vi "tabs_test.vi"() -> ()   [LabVIEW 2015]
panel:
  in  "stop":bool
  in  "Tab Control 2":enum32{"DLTS", "CV", "IV"}(tab)
  in  "Numeric Control":dbl
  in  "Vertical Fill Slide":dbl(slide) scale=0.0..10.0
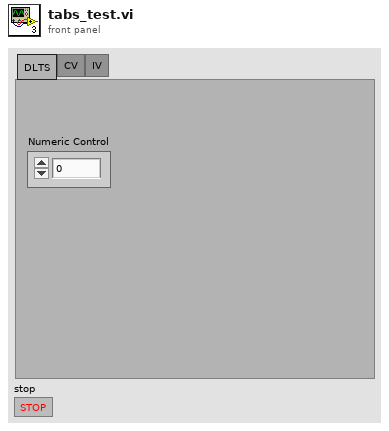
[diagram p1: front panel]
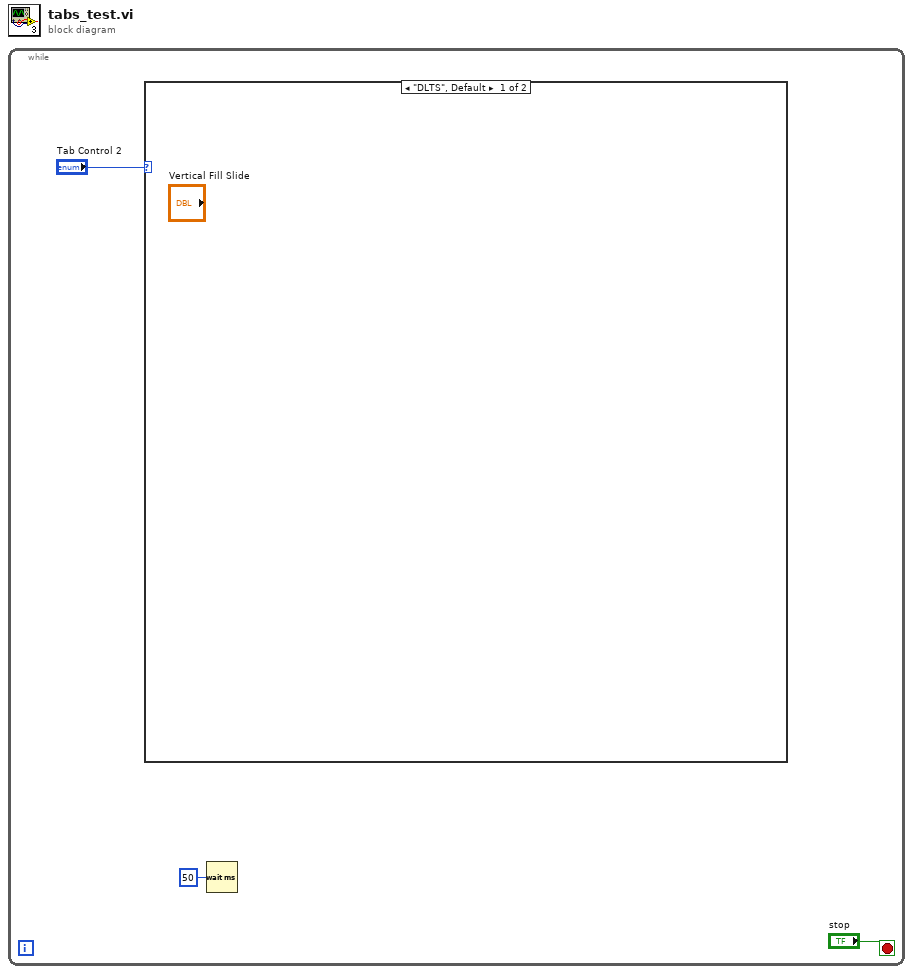
[diagram p0: block diagram]
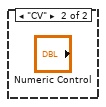
[diagram p2: hidden frame]
diagram:
  n1 = while {
    stop <- "stop" stop-if-true
    n2 = case shown="\"DLTS\", Default" "Tab Control 2" {
      frame "DLTS", Default {
      }
      frame "CV" {
      }
    }
    n3 = Wait (ms)(milliseconds to wait=u32 50) -> ()  [unwired: 1 out]
  }
